vi "mysql_conn.pool_Queue.vi"() -> ()   [LabVIEW 2020]
doc: "该模板用于创建生产者／消费者模式的应用程序。该模板可用于执行诸如数据分析的数据处理，或者在以不均匀速率产生数据的数据源中（如触发采集），当数据可用时对数据进行分析。"
uses:
  <vilib>/addons/database/Connection.llb/Conn ObjectReference.ctl
  <vilib>/addons/database/Connection.llb/Conn Execute.vi
  <vilib>/addons/database/Recordset.llb/Rec Destroy - Connection.vi
  <vilib>/addons/database/Connection.llb/DB Tools Open Connec (String).vi
  <vilib>/addons/database/NI_Database_API.lvlib
panel:
  in  "sql命令数组":string[](array[string])
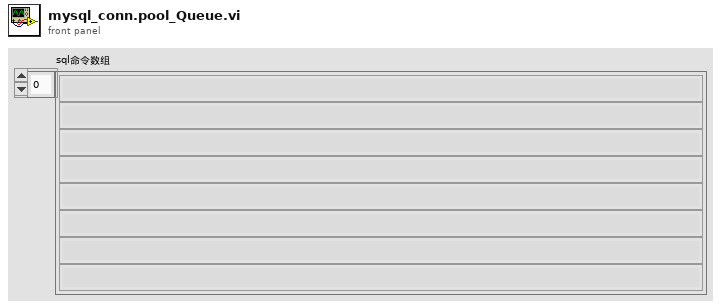
[diagram p1: front panel]
types:
  T1 = typedef "NI_Database_API.lvlib/Conn ObjectReference.ctl" = refnum<k1>
  T2 = typedef "NI_Database_API.lvlib/Rec ObjectReference.ctl" = refnum<k1>
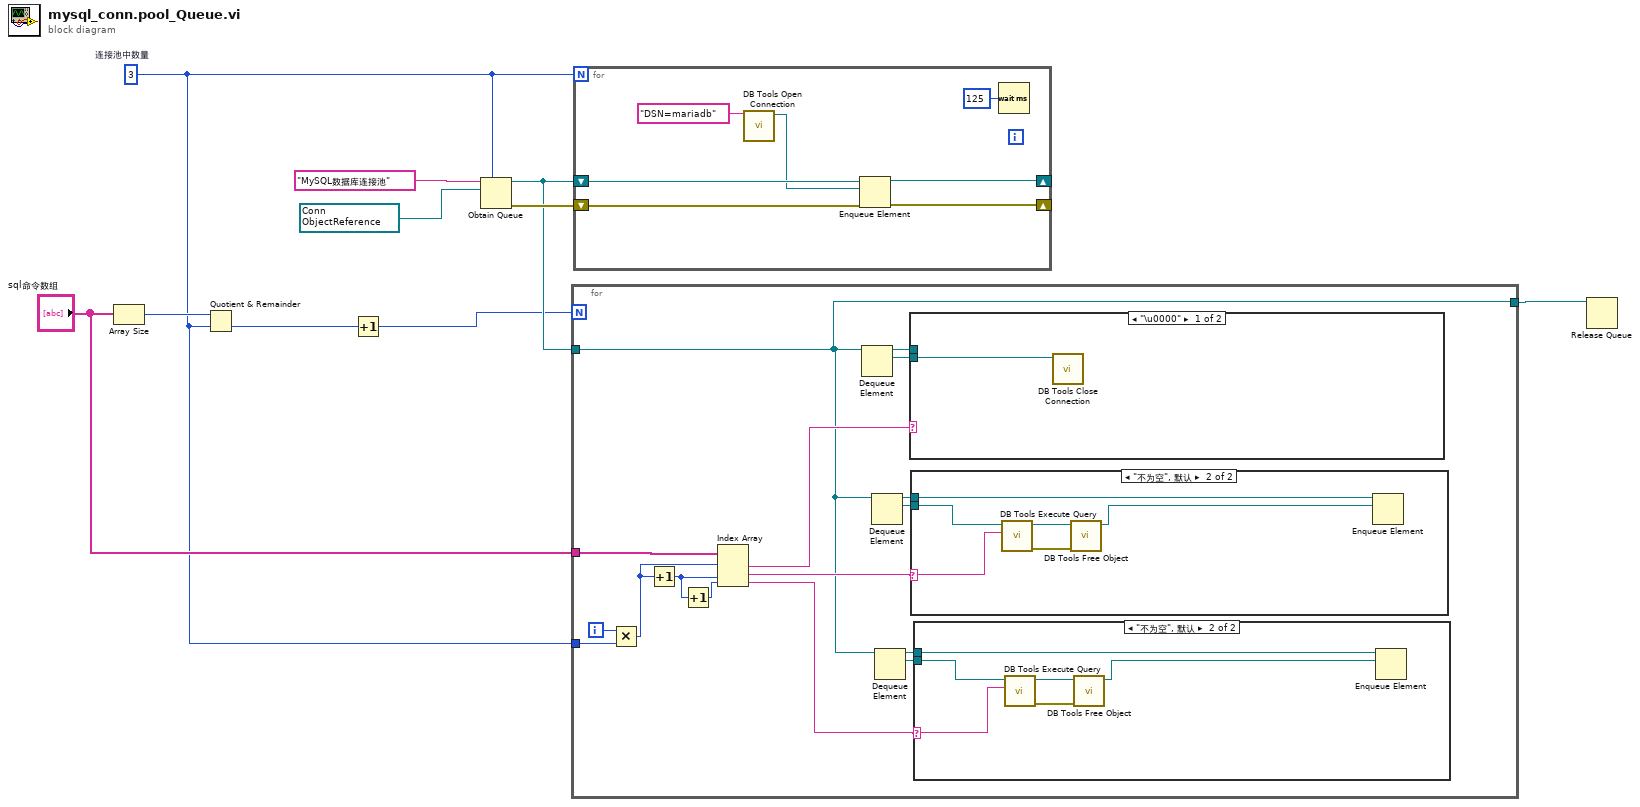
[diagram p0: block diagram]
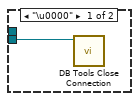
[diagram p2: hidden frame]
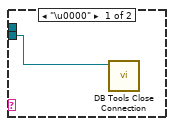
[diagram p3: hidden frame]
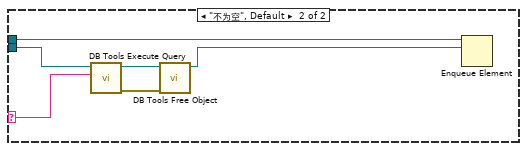
[diagram p4: hidden frame]
diagram:
  w8 = T1 refnum items=["Connection"] ("connection reference")
  w2 = 3  # 连接池中数量
  n1 = Array Size(array="sql命令数组") -> (size(s)=w6:i32)
  n2 = Quotient & Remainder(x=w6, y=w2) -> (floor(x/y)=w5:i32)  [unwired: 1 out]
  n3 = Increment(x=w5) -> (x+1=w4:i32)
  n4 = Obtain Queue(max queue size (-1, unlimited)=w2, name (unnamed)="MySQL数据库连接池" ("名称（未命名）"), element data type=w8) -> (queue out=w7:refnum<queue>, error out=w10:errorcluster)  [unwired: 2 in, 1 out]
  n5 = for {
    N: w4 -> [_]
    tunnel: w7 -> [w11]
    tunnel: "sql命令数组" -> [w20]
    tunnel: w2 -> [w18]
    tunnel: [w11] -> w1
    i -> [w19]
    n6 = Multiply(x=w19, y=w18) -> (x*y=w17:i32)
    n7 = Increment(x=w17) -> (x+1=w15:i32)
    n8 = Increment(x=w15) -> (x+1=w16:i32)
    n9 = Index Array(array=w20, index #1=w17, index #2=w15, index #3=w16) -> (element #1=w14:string, element #2=w13:string, element #3=w12:string)
    n10 = Dequeue Element(queue=w11) -> (queue out=w26:refnum<queue>, element=w25:T1)  [unwired: 2 in, 2 out]
    n11 = Dequeue Element(queue=w11) -> (queue out=w24:refnum<queue>, element=w23:T1)  [unwired: 2 in, 2 out]
    n12 = Dequeue Element(queue=w11) -> (queue out=w22:refnum<queue>, element=w21:T1)  [unwired: 2 in, 2 out]
    n13 = case shown="\"\"" w14 {
      selector: w14 -> [_ w42]
      tunnel: w26 -> [_ w45]
      tunnel: w25 -> [w41 w44]
      frame "\u0000" {
        n14 = call <vilib>:"DB Tools Close Connection.vi"("connection reference"=w41) -> ()  [unwired: 6 in, 1 out]
      }
      frame "不为空", Default {
        n15 = call-poly <vilib>:"DB Tools Execute Query.vi"("SQL query"=w42, "connection reference"=w44) -> ("error out"=w47:errorcluster, "recordset reference"=w46:T2)  [unwired: 6 in]
        n16 = call-poly <vilib>:"DB Tools Free Object.vi"("error in (no error)"=w47, "recordset reference"=w46) -> ("connection reference"=w43:T1)  [unwired: 8 in, 1 out]
        n17 = Enqueue Element(queue=w45, element=w43) -> ()  [unwired: 2 in, 3 out]
      }
    }
    n18 = case shown="\"不为空\", 默认" w13 {
      selector: w13 -> [_ w35]
      tunnel: w24 -> [_ w38]
      tunnel: w23 -> [w34 w37]
      frame "\u0000" {
        n19 = call <vilib>:"DB Tools Close Connection.vi"("connection reference"=w34) -> ()  [unwired: 6 in, 1 out]
      }
      frame "不为空", Default {
        n20 = call-poly <vilib>:"DB Tools Execute Query.vi"("SQL query"=w35, "connection reference"=w37) -> ("error out"=w40:errorcluster, "recordset reference"=w39:T2)  [unwired: 6 in]
        n21 = call-poly <vilib>:"DB Tools Free Object.vi"("error in (no error)"=w40, "recordset reference"=w39) -> ("connection reference"=w36:T1)  [unwired: 8 in, 1 out]
        n22 = Enqueue Element(queue=w38, element=w36) -> ()  [unwired: 2 in, 3 out]
      }
    }
    n23 = case shown="\"不为空\", 默认" w12 {
      selector: w12 -> [_ w28]
      tunnel: w22 -> [_ w31]
      tunnel: w21 -> [w27 w30]
      frame "\u0000" {
        n24 = call <vilib>:"DB Tools Close Connection.vi"("connection reference"=w27) -> ()  [unwired: 6 in, 1 out]
      }
      frame "不为空", Default {
        n25 = call-poly <vilib>:"DB Tools Execute Query.vi"("SQL query"=w28, "connection reference"=w30) -> ("error out"=w33:errorcluster, "recordset reference"=w32:T2)  [unwired: 6 in]
        n26 = call-poly <vilib>:"DB Tools Free Object.vi"("error in (no error)"=w33, "recordset reference"=w32) -> ("connection reference"=w29:T1)  [unwired: 8 in, 1 out]
        n27 = Enqueue Element(queue=w31, element=w29) -> ()  [unwired: 2 in, 3 out]
      }
    }
  }
  n28 = for {
    N: w2 -> [_]
    shift-right: [w51] -> _
    shift-left: w10 -> [w52]
    shift-right: [w53] -> _
    shift-left: w7 -> [w54]
    n29 = call-poly <vilib>:"DB Tools Open Connection.vi"("connection information"="DSN=mariadb") -> ("connection reference"=w48:T1)  [unwired: 7 in, 1 out]
    n30 = Enqueue Element(queue=w54, element=w48, error in (no error)=w52) -> (queue out=w53:refnum<queue>, error out=w51:errorcluster)  [unwired: 1 in, 1 out]
    n31 = Wait (ms)(milliseconds to wait=u32 125) -> ()  [unwired: 1 out]
  }
  n32 = Release Queue(queue=w1) -> ()  [unwired: 2 in, 3 out]
